vi "Image Compute Polygon Interpolated Color.vi"(8 "Decay Range Exponent":dbl=1.0, 9 "1D Color value array":T2(array[cluster]), 10 "Vertices":cluster{"Horizontal":sgl, "Vertical":sgl}[](array[cluster]), 11 "Pixel":T3) -> (1 "Color Components":T1, 3 "Color Value (U32)":u32 format="%.0x")   [LabVIEW 2021, in "Image.lvlib"]
uses:
  Image.lvlib
  <vilib>/vision/NI_Vision_Development_Module.lvlib
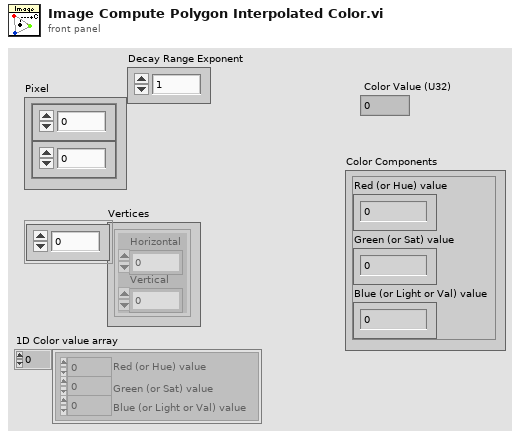
[diagram p1: front panel]
types:
  T1 = cluster{"Red (or Hue) value":u8, "Green (or Sat) value":u8, "Blue (or Light or Val) value":u8}
  T2 = cluster{"Red (or Hue) value":u8, "Green (or Sat) value":u8, "Blue (or Light or Val) value":u8}[]
  T3 = cluster{"Numeric Control":sgl, "Numeric Control":sgl}
  T4 = cluster{"Red (or Hue) value":dbl, "Green (or Sat) value":dbl, "Blue (or Light or Val) value":dbl}
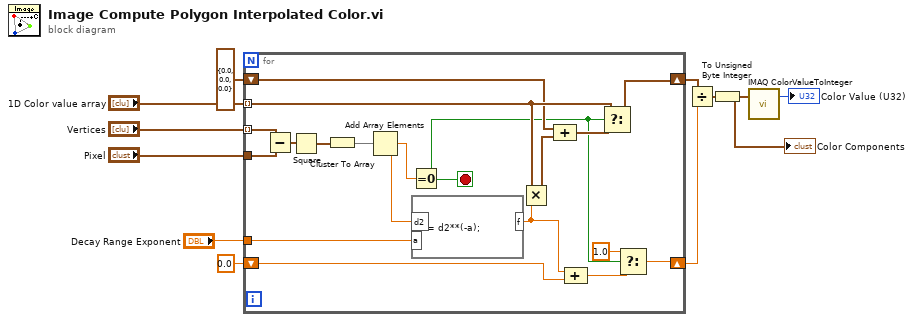
[diagram p0: block diagram]
diagram:
  n1 = for {
    tunnel: "Vertices" -> [w29] mode=indexing
    tunnel: "1D Color value array" -> [w23] mode=indexing
    tunnel: "Pixel" -> [w28]
    shift-right: [w21] -> w6
    shift-left: T4 {"Red (or Hue) value"=0.0, "Green (or Sat) value"=0.0, "Blue (or Light or Val) value"=0.0} ("Color Value") -> [w22]
    shift-right: [w13] -> w5
    shift-left: 0.0 ("t") -> [w16]
    tunnel: "Decay Range Exponent" -> [w12]
    stop <- w18 stop-if-true
    n2 = Subtract(x=w29, y=w28) -> (x-y=w27:cluster{sgl, sgl})
    n3 = Square(x=w27) -> (x^2=w26:cluster{sgl, sgl})
    n4 = Cluster To Array(cluster=w26) -> (array=w25:sgl[])
    n5 = Add Array Elements(numeric array=w25) -> (sum=w24:sgl)
    n6 = Equal To 0?(x=w24) -> (x = 0?=w18:bool)
    n7 = formula code="f = d2**(-a);"("d2"=w24, "a"=w12) -> ("f"=w15:dbl)
    n8 = Multiply(x=w23, y=w15) -> (x*y=w19:T4)
    n9 = Compound Arithmetic op=ADD(w22, w19) -> (w20:T4)
    n10 = Compound Arithmetic op=ADD(w15, w16) -> (w14:dbl)
    n11 = Select(t=w23, s=w18, f=w20) -> (s? t:f=w21:T4)
    n12 = Select(t=1.0, s=w18, f=w14) -> (s? t:f=w13:dbl)
  }
  n13 = Divide(x=w6, y=w5) -> (x/y=w4:T4)
  n14 = To Unsigned Byte Integer(number=w4) -> (unsigned 8bit integer=w2:T1)
  "Color Components" <- w2
  n15 = call "IMAQ ColorValueToInteger"("Color Value"=w2) -> ("U32 value"=→"Color Value (U32)":u32)  [unwired: 4 in, 3 out]
